vi "Override Client Type.vi"(8 "error in (no error)":errorcluster, 11 "HTTP TCP Server in":refnum<class "HTTP TCP Server.lvclass">) -> (0 "error out":errorcluster, 2 "Override Client Type":refnum<class "TCP Client.lvclass">, 3 "HTTP TCP Server out":refnum<class "HTTP TCP Server.lvclass">)   [LabVIEW 2020, in "HTTP Server.lvlib" / "HTTP TCP Server.lvclass"]
uses:
  HTTP TCP Server.lvclass
  <vilib>/IlluminatedG/lv-stream-tcp/TCP Client/TCP Client.lvclass
  HTTP TCP Server.lvclass/HTTP TCP Server.ctl
  HTTP TCP Client/HTTP TCP Client.lvclass
  C:/Program Files (x86)/National Instruments/LabVIEW 2020/vi.lib/IlluminatedG/lv-stream-tcp/TCP Client/TCP Client.lvclass
  C:/Program Files (x86)/National Instruments/LabVIEW 2020/vi.lib/IlluminatedG/lv-stream/Connection/Connection.lvclass
  C:/Program Files (x86)/National Instruments/LabVIEW 2020/vi.lib/IlluminatedG/lv-stream/Endpoint/Endpoint.lvclass
  C:/dev/illuminated-g/lv-http-server/HTTP Server/HTTP TCP Client/HTTP TCP Client.lvclass
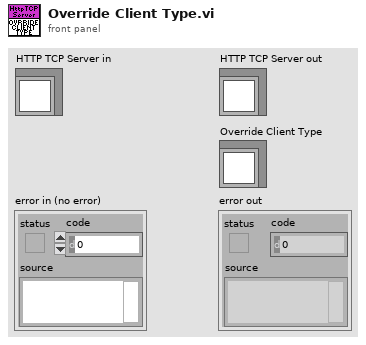
[diagram p1: front panel]
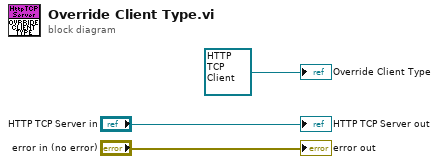
[diagram p0: block diagram]
diagram:
  "error out" <- "error in (no error)"
  "HTTP TCP Server out" <- "HTTP TCP Server in"
  "Override Client Type" <- refnum<class "HTTP TCP Client.lvclass"> refnum ("HTTP Server.lvlib:HTTP TCP Client.lvclass")
